vi "Headless Modular Test W Events.vi"(8 "Core Index (0)":i32, 9 "File Finished Event":refnum<user-event>, 10 "File Status Event":refnum<user-event>, 11 "Path":path) -> ()   [LabVIEW 2018]
uses:
  Classes/Message/Message.lvclass
  Classes/Frame Data Message/Frame Data Message.lvclass
  Classes/STOP Message/STOP.lvclass
  Classes/Video Processor/Video Processor.lvclass
  Classes/Headless Image Processing Handler/Headless Image Processing Handler.lvclass
  49767ad8-b7f6-4460-8d0b-c214da006980.vi
  Video Processor main File Status STYP.ctl
  C:/Users/aaron.jencks/Documents/GitHub/emerson_seed_object_detection/LabVIEW/Projects/Paul's Video Viewer/Classes/Message/Message.lvclass
panel:
  out "Progress":dbl(slide) scale=0.0..100.0
  in  "stop":bool
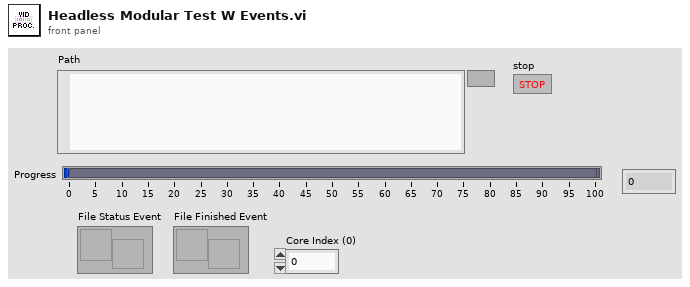
[diagram p1: front panel]
types:
  T1 = typedef "Video Processor main File Status STYP.ctl" = cluster{"Index":i32, "Current Frame":u32, "Total Frames":u32}
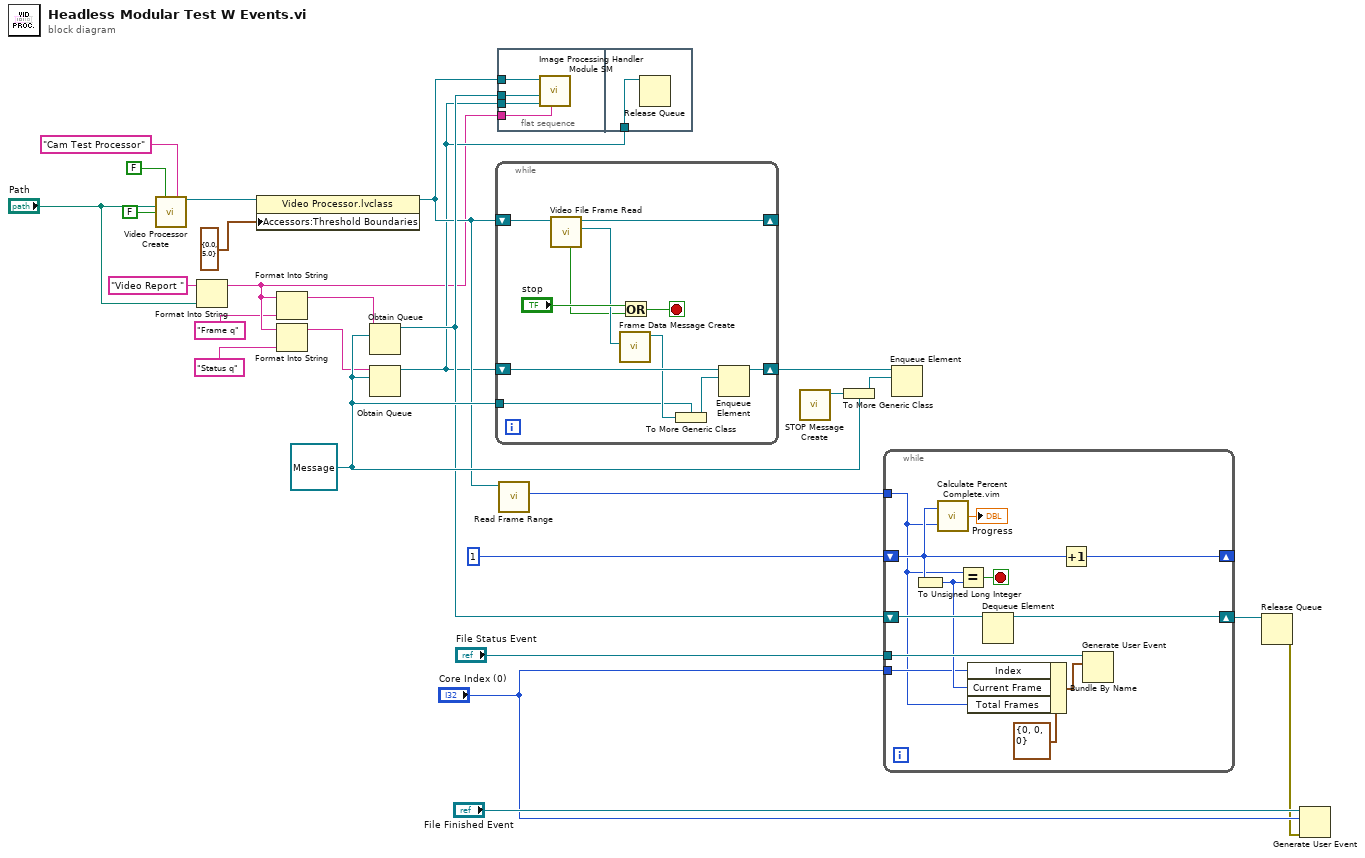
[diagram p0: block diagram]
diagram:
  w18 = refnum<class "Message.lvclass"> refnum ("Message.lvclass")
  n1 = call "Video Processor Create.vi"("Loop? (T)"=FALSE ("Open? (T)"), "Identifier"="Cam Test Processor", "Video Path (\"\")"="Path", "Full? (T)"=FALSE) -> ("Video Processor out"=w20:refnum<class "Video Processor.lvclass">)  [unwired: 10 in, 1 out]
  n2 = Format Into String(initial string="Video Report ", "Path") -> (resulting string=w5:string)  [unwired: 2 in, 1 out]
  n3 = property class="Video Processor.lvclass"(reference=w20, "Accessors:Threshold Boundaries"=cluster{"Minimum":dbl, "Maximum":dbl} {"Minimum"=0.0, "Maximum"=5.0} ("Threshold Boundaries")) -> (reference out=w13:refnum<class "Video Processor.lvclass">)  [unwired: 1 in, 1 out]
  n4 = Format Into String(initial string=w5, "Frame q") -> (resulting string=w2:string)  [unwired: 2 in, 1 out]
  n5 = Format Into String(initial string=w5, "Status q") -> (resulting string=w1:string)  [unwired: 2 in, 1 out]
  n6 = Obtain Queue(name (unnamed)=w2, element data type=w18) -> (queue out=w15:refnum<queue>)  [unwired: 3 in, 2 out]
  n7 = Obtain Queue(name (unnamed)=w1, element data type=w18) -> (queue out=w6:refnum<queue>)  [unwired: 3 in, 2 out]
  n8 = while {
    shift-right: [w27] -> _
    shift-left: w13 -> [w37]
    tunnel: w18 -> [w32]
    shift-right: [w30] -> w26
    shift-left: w6 -> [w34]
    stop <- w29 stop-if-true
    n9 = call-dynamic "Video File Frame Read.vi"("Video Processor in"=w37) -> ("Video Frame out"=w35:refnum<class "Video Frame.lvclass">, "Video Processor out"=w27:refnum<class "Video Processor.lvclass">, "Playback Finished?"=w28:bool)  [unwired: 6 in, 2 out]
    n10 = call "Frame Data Message Create.vi"("Video Frame"=w35) -> ("Frame Data Message out"=w33:refnum<class "Frame Data Message.lvclass">)  [unwired: 9 in, 1 out]
    n11 = Or(x="stop", y=w28) -> (x .or. y?=w29:bool)
    n12 = To More Generic Class(target class=w32, reference=w33) -> (generic class reference=w31:refnum<class "Message.lvclass">)
    n13 = Enqueue Element(queue=w34, element=w31) -> (queue out=w30:refnum<queue>)  [unwired: 2 in, 2 out]
  }
  n14 = flat-sequence {
    tunnel: w6 -> [w41]
    tunnel: w5 -> [w40]
    tunnel: w15 -> [w39]
    tunnel: w13 -> [w38]
    tunnel: w6 -> [w42]
    frame #0 {
      n15 = call "Image Processing Handler Module SM.vi"("Identifier"=w40, "data queue"=w41, "tx data queue"=w39, "Video Processor"=w38) -> ()  [unwired: 8 in]
    }
    frame #1 {
      n16 = Release Queue(queue=w42) -> ()  [unwired: 2 in, 3 out]
    }
  }
  n17 = call-dynamic "Read Frame Range.vi"("Video File in"=w13) -> ("Number of Frames"=w12:u32)  [unwired: 8 in, 2 out]
  n18 = call "STOP Message Create.vi"() -> ("STOP out"=w25:refnum<class "STOP.lvclass">)  [unwired: 10 in, 1 out]
  n19 = To More Generic Class(target class=w18, reference=w25) -> (generic class reference=w24:refnum<class "Message.lvclass">)
  n20 = while {
    shift-right: [w53] -> w8
    shift-left: w15 -> [w54]
    shift-right: [w52] -> _
    shift-left: 1 -> [w44]
    tunnel: w12 -> [w43]
    tunnel: "File Status Event" -> [w49]
    tunnel: "Core Index (0)" -> [w45]
    stop <- w50 stop-if-true
    n21 = To Unsigned Long Integer(number=w44) -> (unsigned 32bit integer=w46:u32)
    n22 = call "Calculate Percent Complete.vim"("Total"=w43, "Part"=w44) -> ("% Complete"=→"Progress":dbl)
    n23 = Equal?(x=w43, y=w46) -> (x = y?=w50:bool)
    n24 = Bundle By Name(cluster=T1 {"Index"=0, "Current Frame"=0, "Total Frames"=0} ("event data"), "Index"=w45, "Current Frame"=w46, "Total Frames"=w43) -> (w47:T1)
    n25 = Dequeue Element(queue=w54) -> (queue out=w53:refnum<queue>)  [unwired: 2 in, 3 out]
    n26 = Increment(x=w44) -> (x+1=w52:i32)
    n27 = Generate User Event(user event=w49, event data cluster=w47) -> ()  [unwired: 2 in, 2 out]
  }
  n28 = Enqueue Element(queue=w26, element=w24) -> ()  [unwired: 2 in, 3 out]
  n29 = Release Queue(queue=w8) -> (error out=w7:errorcluster)  [unwired: 2 in, 2 out]
  n30 = Generate User Event(user event="File Finished Event", event data cluster="Core Index (0)", error in=w7) -> ()  [unwired: 1 in, 2 out]
